vi "Toggle.vi"(1 "Input":bool) -> (0 "Output":bool)   [LabVIEW 2014]
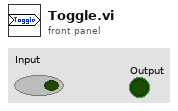
[diagram p1: front panel]
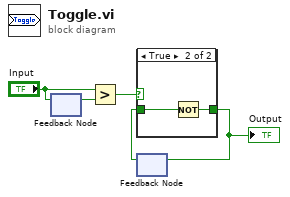
[diagram p0: block diagram]
diagram:
  n1 = feedback-in #1("Input") -> ()
  n2 = feedback #1() -> (w4:bool)  [unwired: 1 in]
  n3 = Greater?(x="Input", y=w4) -> (0:w3:bool)
  n4 = feedback #2() -> (w1:bool)  [unwired: 1 in]
  n5 = case shown="True" w3 {
    tunnel: [w6 w8] -> w2
    tunnel: w1 -> [w6 w7]
    frame False {
    }
    frame True {
      n6 = Not(x=w7) -> (.not. x?=w8:bool)
    }
  }
  "Output" <- w2
  n7 = feedback-in #2(w2) -> ()
